vi "test transactions.vi"() -> ()   [LabVIEW 2023]
uses:
  Database.lvlib
panel:
  in  "port":i32=3306
  in  "host":string="localhost"
  in  "password":string="carriker"
  in  "username":string="root"
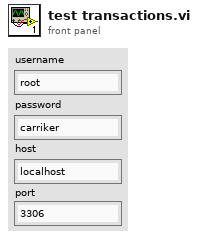
[diagram p1: front panel]
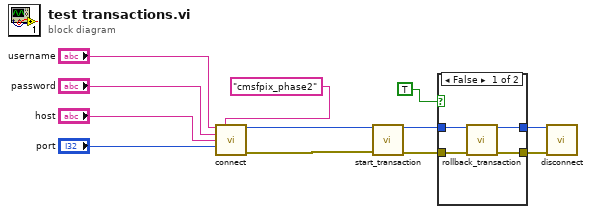
[diagram p0: block diagram]
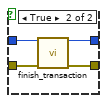
[diagram p2: hidden frame]
diagram:
  n1 = call "connect.vi"("username"="username", "schema"="cmsfpix_phase2" ("Schema"), "password"="password", "host"="host", "port"="port") -> ("DB Session ID"=w7:i32, "error out"=w6:errorcluster)  [unwired: 9 in]
  n2 = call "start_transaction.vi"("DB Session ID"=w7, "error in (no error)"=w6) -> ("DB Session ID out"=w5:i32, "error out"=w4:errorcluster)  [unwired: 12 in]
  n3 = case shown="False" TRUE {
    tunnel: w5 -> [w16 w20]
    tunnel: w4 -> [w14 w19]
    tunnel: [w15 w18] -> w3
    tunnel: [w13 w17] -> w2
    frame False {
      n4 = call "rollback_transaction.vi"("DB Session ID"=w16, "error in (no error)"=w14) -> ("DB Session ID out"=w15:i32, "error out"=w13:errorcluster)  [unwired: 12 in]
    }
    frame True {
      n5 = call "finish_transaction.vi"("DB Session ID"=w20, "error in (no error)"=w19) -> ("DB Session ID out"=w18:i32, "error out"=w17:errorcluster)  [unwired: 12 in]
    }
  }
  n6 = call "disconnect.vi"("DB Session ID"=w3, "error in (no error)"=w2) -> ()  [unwired: 13 in, 1 out]
